vi "AWG_Initialization.vi"(8 "error in (no error)":errorcluster, 10 "AWG Parameters":T2[](array[typedef]) {"Value" format="%#_6p"}, 11 "Address":string) -> (0 "error out":errorcluster, 2 "Selected Device":string, 3 "AWG Handle Out":T1 {"Handle" format="0x%08x"; "Conn" format="0x%08x"})   [LabVIEW 2016, in "ZI AWG.lvlib"]
uses:
  ZI AWG.lvlib
  Ctl_SetParameter(Value).ctl
  <instrlib>/Zurich Instruments LabOne/Public/ziTypeHandle.ctl
  <instrlib>/Zurich Instruments LabOne/Zurich Instruments LabOne.lvlib
  General.lvlib
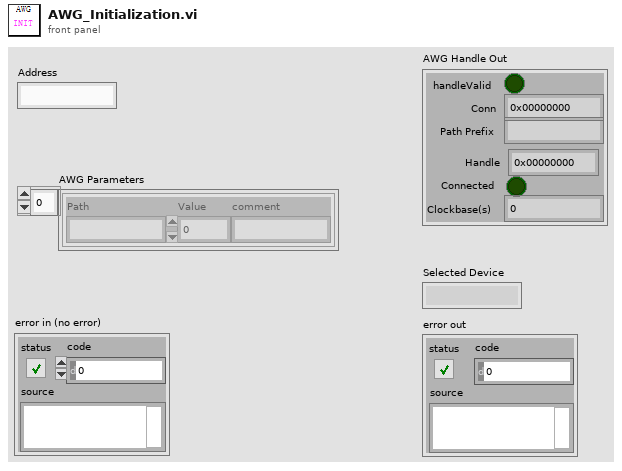
[diagram p1: front panel]
types:
  T1 = typedef "Zurich Instruments LabOne.lvlib/ziTypeHandle.ctl" = cluster{"handleValid":bool, "Conn":u64, "Path Prefix":string, "Handle":u64, "Connected":bool, "Clockbase(s)":dbl}
  T2 = typedef "General.lvlib/Ctl_SetParameter(Value).ctl" = cluster{"Path":string, "Value":dbl, "comment":string}
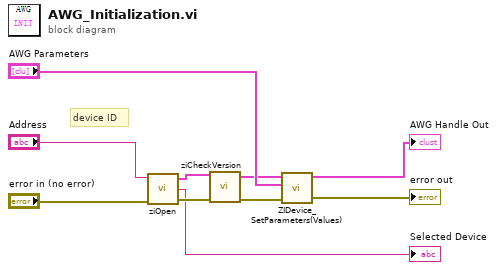
[diagram p0: block diagram]
diagram:
  # "device ID"
  n1 = call <instrlib>:"ziOpen.vi"("Error In"="error in (no error)", "Address"="Address") -> ("Error Out"=w6:errorcluster, "Selected Device"=→"Selected Device":string, "HandleOut"=w8:T1)  [unwired: 2 out]
  n2 = call <instrlib>:"ziCheckVersion.vi"("Handle In"=w8, "Error In"=w6) -> ("Handle Out"=w1:T1, "Error Out"=w7:errorcluster)  [unwired: 11 in, 1 out]
  n3 = call "ZIDevice_SetParameters(Values).vi"("error in (no error)"=w7, "Parameters"="AWG Parameters", "Handle In"=w1) -> ("error out"=→"error out":errorcluster, "Handle Out"=→"AWG Handle Out":T1)  [unwired: 7 in]
